vi "无边框窗口-拖动窗口.vi"() -> ()   [LabVIEW 2013]
uses:
  <vilib>/Utility/miscctls.llb/LVPointTypeDef.ctl
  <vilib>/Utility/miscctls.llb/LVPoint32TypeDef.ctl
panel:
  in  "菜单下拉列表":u16(ring)
  in  "按下时鼠标坐标":T1 caption="坐标"
  out "窗格-鼠标按下？":bool=TRUE
  in  "停止按钮":bool
  out "类型":T2(ring)
  out "前面板窗口:最小尺寸":T3
  out "前面板窗口:动作":T4(ring)
  out "项标识符":string
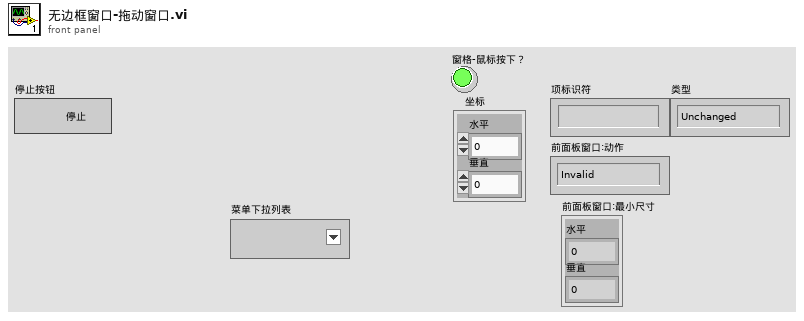
[diagram p1: front panel]
types:
  T1 = typedef "LVPoint32TypeDef.ctl" = cluster{"Horizontal":i32, "Vertical":i32}
  T2 = enum32{"Unchanged", "Centered", "Maximized", "Minimized", "Custom"}
  T3 = typedef "LVPointTypeDef.ctl" = cluster{"Horizontal":i16, "Vertical":i16}
  T4 = enum32{"Invalid", "Default", "Floating", "Floating/Auto-Hide", "Modal"}
  T5 = typedef "LVRectTypeDef.ctl" = cluster{"Left":i16, "Top":i16, "Right":i16, "Bottom":i16}
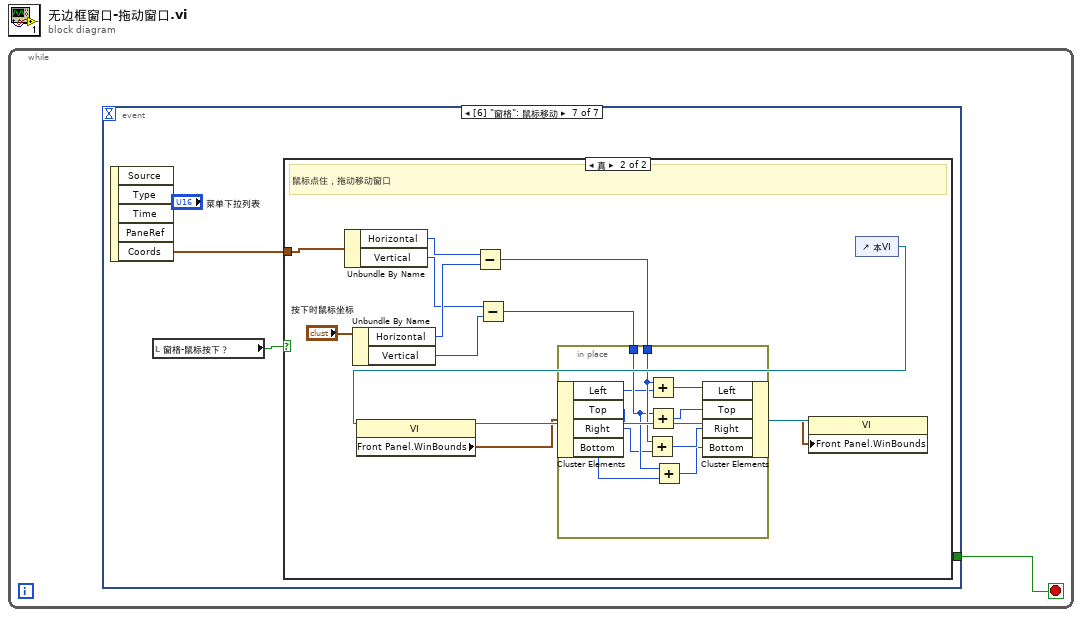
[diagram p0: block diagram]
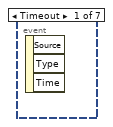
[diagram p2: hidden frame]
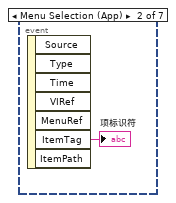
[diagram p3: hidden frame]
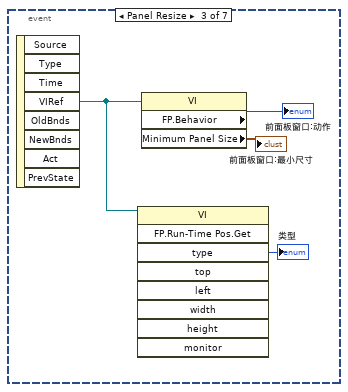
[diagram p4: hidden frame]
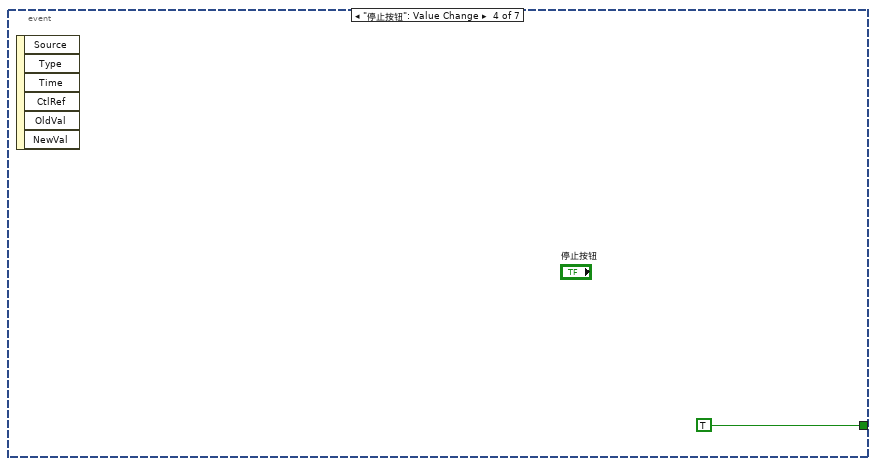
[diagram p5: hidden frame]
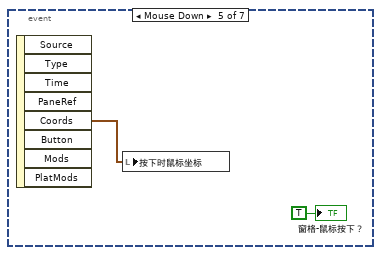
[diagram p6: hidden frame]
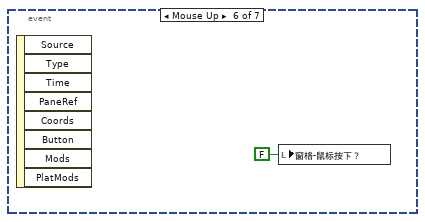
[diagram p7: hidden frame]
diagram:
  n1 = while {
    stop <- w1 stop-if-true
    n2 = event shown="[6] \"窗格\": 鼠标移动" {
      selector: _ -> [_ _ _ _ _ _ _]
      dyn-events: _ -> [_ _ _ _ _ _ _]
      timeout: _ -> [_ _ _ _ _ _ _]
      tunnel: [_ _ _ TRUE ("停止按钮") _ _ _] -> w1
      event Timeout {
        n3 = event-data() -> ()  [unwired: 1 in, 3 out]
      }
      event Menu Selection (App) {
        n4 = event-data() -> ("ItemTag"=→"项标识符":string)  [unwired: 1 in, 6 out]
      }
      event Panel Resize {
        n5 = event-data() -> ("VIRef"=w4:refnum<vi>)  [unwired: 1 in, 7 out]
        n6 = invoke class="VI" method="FP.Run-Time Pos.Get"(reference=w4) -> ("type"=→"类型":T2)  [unwired: 8 in, 8 out]
        n7 = property class="VI"(reference=w4) -> ("FP.Behavior"=→"前面板窗口:动作":T4, "Minimum Panel Size"=→"前面板窗口:最小尺寸":T3)  [unwired: 1 in, 2 out]
      }
      event "停止按钮": Value Change {
        n8 = event-data() -> ()  [unwired: 1 in, 6 out]
      }
      event Mouse Down {
        n9 = event-data() -> ("Coords"=w8:T1)  [unwired: 1 in, 7 out]
        n10 = local write "按下时鼠标坐标"(w8) -> ()
        "窗格-鼠标按下？" <- TRUE ("窗格-鼠标按下？")
      }
      event Mouse Up {
        n11 = event-data() -> ()  [unwired: 1 in, 8 out]
        n12 = local write "窗格-鼠标按下？"(FALSE ("窗格-鼠标按下？")) -> ()
      }
      event Mouse Move {
        n13 = event-data() -> ("Coords"=w11:T1)  [unwired: 1 in, 4 out]
        n14 = local read "窗格-鼠标按下？"() -> (w12:bool)
        n15 = case shown="真" w12 {
          tunnel: w11 -> [_ w23]
          frame False {
          }
          frame True {
            # "鼠标点住，拖动移动窗口"
            n16 = Unbundle By Name(w23) -> ("Horizontal"=w22:i32, "Vertical"=w20:i32)
            n17 = Unbundle By Name("按下时鼠标坐标") -> ("Horizontal"=w21:i32, "Vertical"=w19:i32)
            n18 = Subtract(x=w22, y=w21) -> (x-y=w15:i32)
            n19 = Subtract(x=w20, y=w19) -> (x-y=w14:i32)
            n20 = control-ref of="本VI"() -> (w18:refnum<vi>)
            n21 = property class="VI"(reference=w18) -> (reference out=w17:refnum<vi>, "Front Panel.WinBounds"=w16:T5)  [unwired: 1 in, 1 out]
            n22 = in-place {
              in-place-border: w15 -> [w34]
              in-place-border: w14 -> [w33]
              n23 = in-place-cluster #1(w16) -> ("Left"=w32:i16, "Top"=w31:i16, "Right"=w30:i16, "Bottom"=w29:i16)
              n24 = Add(x=w34, y=w30) -> (x+y=w26:i32)
              n25 = Add(x=w34, y=w32) -> (x+y=w28:i32)
              n26 = Add(x=w33, y=w31) -> (x+y=w27:i32)
              n27 = Add(x=w33, y=w29) -> (x+y=w25:i32)
              n28 = in-place-cluster #1("Left"=w28, "Top"=w27, "Right"=w26, "Bottom"=w25) -> (w13:T5)
            }
            n29 = property class="VI"(reference=w17, "Front Panel.WinBounds"=w13) -> ()  [unwired: 1 in, 2 out]
          }
        }
      }
    }
  }
